vi "Read Configuration OO-DB.vi"() -> ()   [LabVIEW 2016, in "DB-Configuration.lvlib"]
doc: "Read object oriented configuration data from database using the configuration class.\n\nLizenziert unter EUPL V. 1.1"
uses:
  DB-Configuration.lvlib
  Configuration/Classes/Configuration/Configuration.lvclass
  ODBC-Interface/ODBC-Interface.lvclass
  C:/User/Brand/LVP/VIP2012/Configuration/Classes/Interface/Interface.lvclass
panel:
  in  "password":string
  in  "userID":string="postgres"
  in  "connection information":string="PostgreSQL30"
  out "Sections":T1(array[cluster])
  out "Configuration out":refnum<class "Configuration.lvclass">
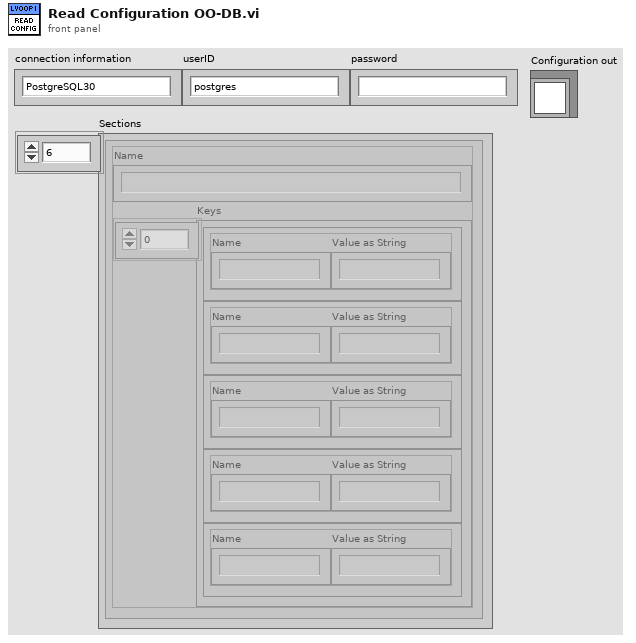
[diagram p1: front panel]
types:
  T1 = cluster{"Name":string, "Keys":cluster{"Name":string, "Value as String":string}[]}[]
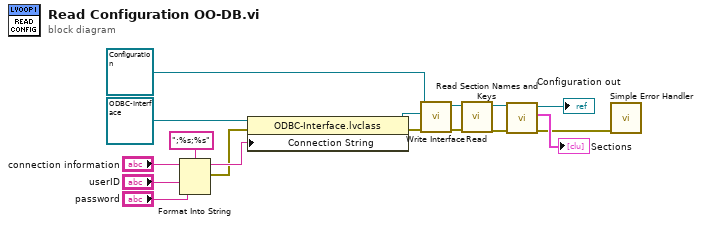
[diagram p0: block diagram]
diagram:
  n1 = Format Into String(format string=";%s;%s", initial string="connection information", "userID", "password") -> (resulting string=w4:string, error out=w3:errorcluster)  [unwired: 1 in]
  n2 = property class="ODBC-Interface.lvclass"(reference=refnum<class "ODBC-Interface.lvclass"> refnum ("DB-Configuration.lvlib:ODBC-Interface.lvclass"), error in=w3, "Connection String"=w4) -> (reference out=w13:refnum<class "ODBC-Interface.lvclass">, error out=w16:errorcluster)
  n3 = call "Write Interface.vi"("error in (no error)"=w16, "Interface"=w13, "Configuration in"=refnum<class "Configuration.lvclass"> refnum) -> ("error out"=w15:errorcluster, "Configuration out"=w14:refnum<class "Configuration.lvclass">)  [unwired: 7 in]
  n4 = call "Read.vi"("error in (no error)"=w15, "Configuration"=w14) -> ("error out"=w1:errorcluster, "Configuration out"=w2:refnum<class "Configuration.lvclass">)  [unwired: 8 in]
  n5 = call "Read Section Names and Keys.vi"("error in (no error)"=w1, "Configuration in"=w2) -> ("error out"=w11:errorcluster, "Sections"=→"Sections":T1, "Configuration out"=→"Configuration out":refnum<class "Configuration.lvclass">)  [unwired: 7 in]
  n6 = call <vilib>:"Simple Error Handler.vi"("error in (no error)"=w11) -> ()  [unwired: 4 in, 5 out]
